vi "PM100D_GetRngLbl.vi"(3 "PM16":bool, 4 "MainUnits":enum16{"W", "V", "J", "dBm", "A"}(ring), 5 "PM100D":refnum<visa-resource-name>) -> (0 "Auto":bool, 1 "Numeric":dbl, 2 "String":string)   [LabVIEW 2011]
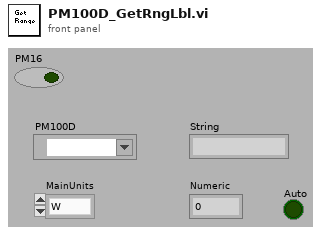
[diagram p1: front panel]
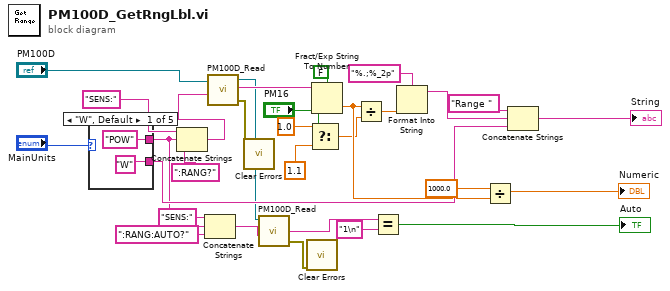
[diagram p0: block diagram]
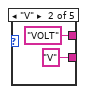
[diagram p2: hidden frame]
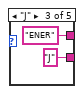
[diagram p3: hidden frame]
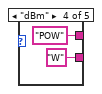
[diagram p4: hidden frame]
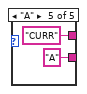
[diagram p5: hidden frame]
diagram:
  n1 = case shown="\"W\", Default" "MainUnits" {
    tunnel: ["POW" "VOLT" "ENER" "POW" "CURR"] -> w12
    tunnel: ["W" "V" "J" "W" "A"] -> w28
    frame "W", Default {
    }
    frame "V" {
    }
    frame "J" {
    }
    frame "dBm" {
    }
    frame "A" {
    }
  }
  n2 = Concatenate Strings("SENS:" ("string"), w12, ":RANG?" ("string")) -> (w26:string)
  n3 = Concatenate Strings("SENS:" ("string"), w12, ":RANG:AUTO?" ("string")) -> (w10:string)
  n4 = call "PM100D_Read.vi"("Command"=w26, "VISA in"="PM100D") -> ("error out"=w15:errorcluster, "ReadValue"=w19:string, "VISA out"=w14:refnum<visa-resource-name>)  [unwired: 2 in]
  n5 = call <vilib>:"Clear Errors.vi"("error in (no error)"=w15) -> ()  [unwired: 6 in, 1 out]
  n6 = call "PM100D_Read.vi"("Command"=w10, "VISA in"=w14) -> ("error out"=w13:errorcluster, "ReadValue"=w9:string)  [unwired: 2 in, 1 out]
  n7 = call <vilib>:"Clear Errors.vi"("error in (no error)"=w13) -> ()  [unwired: 6 in, 1 out]
  n8 = Select(t=1.0, s="PM16", f=1.1 ("y")) -> (s? t:f=w2:dbl)
  n9 = Fract/Exp String To Number(use system decimal point (T)=FALSE, string=w19) -> (number=w24:dbl)  [unwired: 2 in, 1 out]
  n10 = Divide(x=w24, y=w2) -> (x/y=w17:dbl)
  n11 = Equal?(x=w9, y="1\n") -> (x = y?=→"Auto":bool)
  n12 = Format Into String(format string="%.;%_2p", w17) -> (resulting string=w29:string)  [unwired: 2 in, 1 out]
  n13 = Divide(x=1000.0, y=w24) -> (x/y=→"Numeric":dbl)
  n14 = Concatenate Strings("Range " ("string"), w29, w28) -> (→"String":string)
